vi "Send Control Drag Source Update.vi"(0 "Message Enqueuer in":refnum<class "Message Enqueuer.lvclass">, 3 "EventFilter Reference":T1, 5 "CtlRef":refnum<vi>, 7 "Time":u32, 9 "Result":enum16{"Drop Cancel", "Drop Move", "Drop Copy"}(ring)) -> (4 "Filtered EventDataMessage":refnum<class "ControlDragSourceUpdateMsg.lvclass">, 15 "error out":errorcluster)   [LabVIEW 2017, in "ActorEvents.lvlib" / "ControlDragSourceUpdateMsg.lvclass"]
doc: "<License>\nCopyright © 2017 Composed Systems, LLC | All rights reserved\nwww.composed.io\n\nAuthor: Ethan Stern <ethan.stern@composed.io>\n\nThis software is provided \"AS IS\" WITHOUT WARRANTIES, either express or implied, AND IS FOR EDUCATIONAL PURPOSES ONLY.\n</License>"
uses:
  ControlDragSourceUpdateMsg.lvclass
  <vilib>/ActorFramework/Message Enqueuer/Message Enqueuer.lvclass
  c:/Git/mva-viewable/Source/ActorEvents/IEventAggregator Messages/EventDataMessage/EventDataMessage.lvclass
  IEventFilter/EventFilter Reference.ctl
  IEventFilter/IEventFilter.lvclass
  ControlDragSourceUpdateMsg.lvclass/ControlDragSourceUpdateMsg.ctl
  EventDataMessage/EventDataMessage.lvclass/EventDataMessage.ctl
  <vilib>/ActorFramework/Message Enqueuer/Message Enqueuer.lvclass/Message Enqueuer.ctl
  <vilib>/ActorFramework/Message Enqueuer/Enqueue.vi
  <vilib>/Utility/error.llb/Clear Errors.vi
  EventDataMessage/EventDataMessage.lvclass
  C:/Program Files (x86)/National Instruments/LabVIEW 2017/vi.lib/ActorFramework/Message/Message.lvclass
  <vilib>/ActorFramework/Message Priority Queue/Priority Enqueue.vi
panel:
  in  "error in (no error)":errorcluster
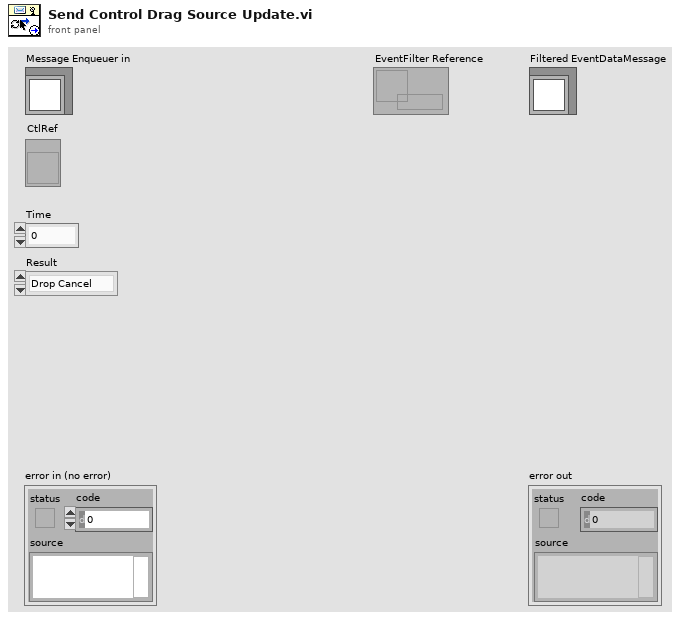
[diagram p1: front panel]
types:
  T1 = typedef "ActorEvents.lvlib/IEventFilter.lvclass/EventFilter Reference.ctl" = refnum<data-value>
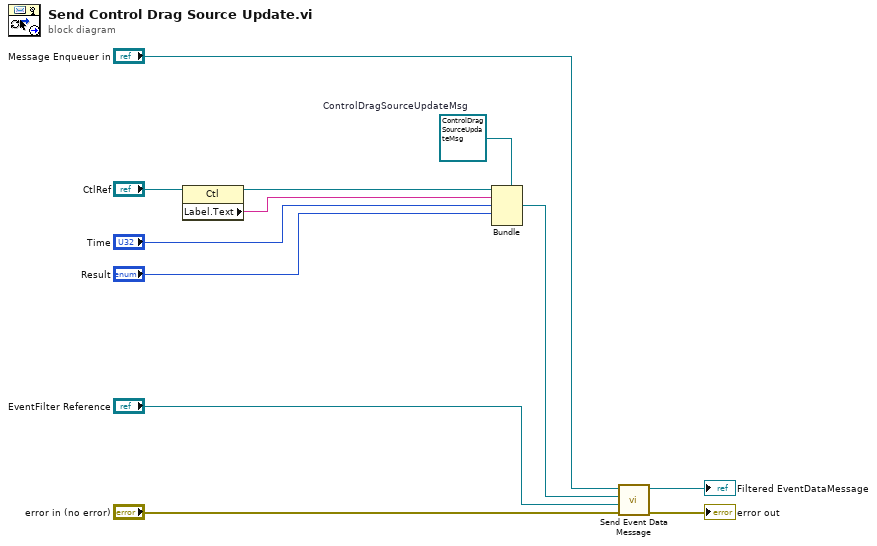
[diagram p0: block diagram]
diagram:
  w12 = refnum<class "ControlDragSourceUpdateMsg.lvclass"> refnum  # ControlDragSourceUpdateMsg
  n1 = property class="Ctl"(reference="CtlRef") -> (reference out=w6:refnum<vi>, "Label.Text"=w5:string)  [unwired: 1 in, 1 out]
  n2 = Bundle(cluster=w12, w6, w5, "Time", "Result") -> (w9:refnum<class "ControlDragSourceUpdateMsg.lvclass">)  [unwired: 1 in]
  n3 = call "Send Event Data Message.vi"("error in (no error)"="error in (no error)", "EventFilter Reference"="EventFilter Reference", "EventDataMessage"=w9, "Message Enqueuer in"="Message Enqueuer in") -> ("error out"=→"error out":errorcluster, "Filtered EventDataMessage"=→"Filtered EventDataMessage":refnum<class "ControlDragSourceUpdateMsg.lvclass">)  [unwired: 6 in]
